vi "NewHttpSession.vi"(8 "error in":errorcluster, 11 "base url":string) -> (0 "error out":errorcluster, 3 "reQwestClient":refnum<class "reQwestClient.lvclass">)   [LabVIEW 2020, in "reQwestClient.lvclass"]
uses:
  reQwestClient.lvclass
  reQwestClient.lvclass/reQwestClient.ctl
  submodules/reqwest-rs-labview/lv_src/ClientBuilder/ClientBuilder.lvclass
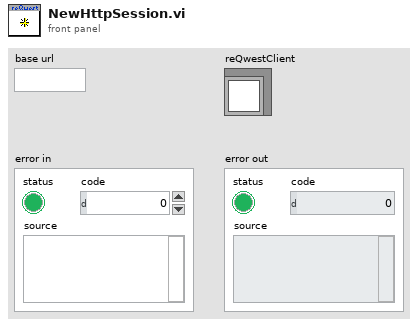
[diagram p1: front panel]
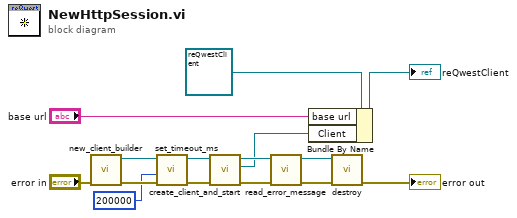
[diagram p0: block diagram]
diagram:
  n1 = call "new_client_builder.vi"("error in (no error)"="error in") -> ("error out"=w6:errorcluster, "Client out"=w5:refnum<class "ClientBuilder.lvclass">)  [unwired: 9 in]
  n2 = call "set_timeout_ms.vi"("error in (no error)"=w6, "timeout_secs"=u64 200000, "ClientBuilder in"=w5) -> ("error out"=w4:errorcluster, "ClientBuilder out"=w3:refnum<class "ClientBuilder.lvclass">)  [unwired: 6 in, 1 out]
  n3 = call "create_client_and_start.vi"("error in"=w4, "ClientBuilder in"=w3) -> ("error out"=w13:errorcluster, "Client out"=w9:refnum<class "Client.lvclass">, "ClientBuilder out"=w15:refnum<class "ClientBuilder.lvclass">)  [unwired: 7 in]
  n4 = call "read_error_message.vi"("error in (no error)"=w13, "ClientBuilder in"=w15) -> ("error out"=w12:errorcluster, "ClientBuilder in"=w14:refnum<class "ClientBuilder.lvclass">)  [unwired: 7 in, 1 out]
  n5 = Bundle By Name(cluster=refnum<class "reQwestClient.lvclass"> refnum ("reQwestClient out"), "base url"="base url", "Client"=w9) -> (→"reQwestClient":refnum<class "reQwestClient.lvclass">)
  n6 = call "destroy.vi"("error in (no error)"=w12, "ClientBuilder in"=w14) -> ("error out"=→"error out":errorcluster)  [unwired: 9 in]
